vi "Check Inhibit.vi"(8 "error in (no error)":errorcluster, 11 "Element Inhibit in":refnum<class "Element Inhibit.lvclass">) -> (0 "error out":errorcluster, 3 "Element Inhibit out":refnum<class "Element Inhibit.lvclass">)   [LabVIEW 2020, in "VolatusGUI.lvlib" / "Element Inhibit.lvclass"]
uses:
  Element Inhibit.lvclass
  Element Inhibit.lvclass/Element Inhibit.ctl
  lv-vecto/Vecto/Channel DBL/Channel DBL.lvclass
  lv-vecto/Vecto/Vecto.lvlib
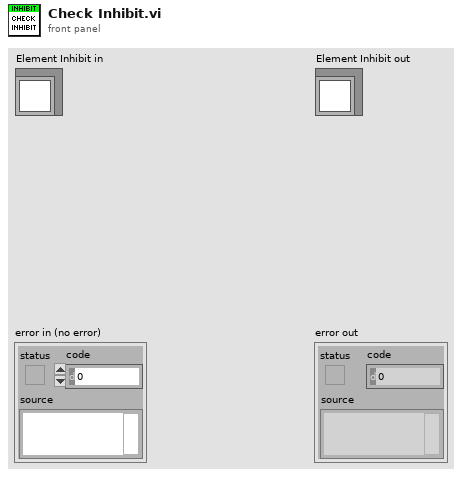
[diagram p1: front panel]
types:
  T1 = enum8{"Enabled", "Disabled", "Disabled and Grayed Out"}
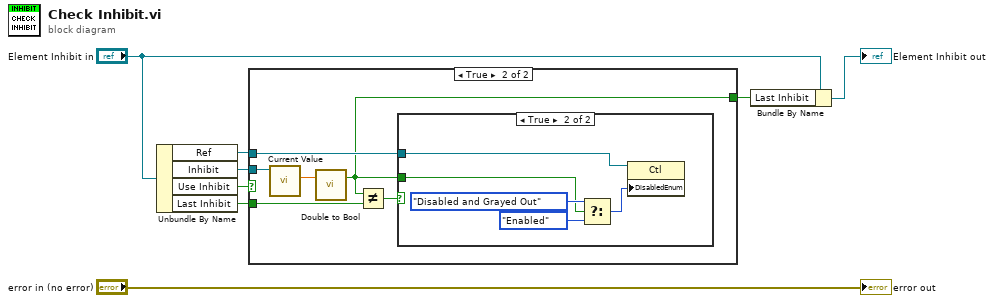
[diagram p0: block diagram]
diagram:
  n1 = Unbundle By Name("Element Inhibit in") -> ("Ref"=w3:refnum<vi>, "Inhibit"=w5:refnum<class "Channel DBL.lvclass">, "Use Inhibit"=w6:bool, "Last Inhibit"=w4:bool)
  n2 = case shown="True" w6 {
    tunnel: w5 -> [_ w15]
    tunnel: w4 -> [w9 w13]
    tunnel: w3 -> [_ w11]
    tunnel: [w9 w10] -> w1
    frame False {
    }
    frame True {
      n3 = call "Current Value.vi"("Channel in"=w15) -> ("Scaled"=w14:dbl)  [unwired: 6 in, 4 out]
      n4 = call "Double to Bool.vi"("Double"=w14) -> ("Bool"=w10:bool)  [unwired: 2 in]
      n5 = Not Equal?(x=w10, y=w13) -> (x != y?=w12:bool)
      n6 = case shown="True" w12 {
        tunnel: w10 -> [_ w17]
        tunnel: w11 -> [_ w16]
        frame False {
        }
        frame True {
          n7 = Select(t=T1."Disabled and Grayed Out" ("Disabled"), s=w17, f=T1."Enabled" ("Disabled")) -> (s? t:f=w18:T1)
          n8 = property class="Ctl"(reference=w16, "DisabledEnum"=w18) -> ()  [unwired: 1 in, 2 out]
        }
      }
    }
  }
  n9 = Bundle By Name(cluster="Element Inhibit in", "Last Inhibit"=w1) -> (→"Element Inhibit out":refnum<class "Element Inhibit.lvclass">)
  "error out" <- "error in (no error)"
